vi "LEDName2Counter.vi"(10 "LED Name":string, 11 "LED Values":T1(array[cluster])) -> (3 "Counter":string)   [LabVIEW 2010, in "Settings.lvclass"]
uses:
  Settings.lvclass
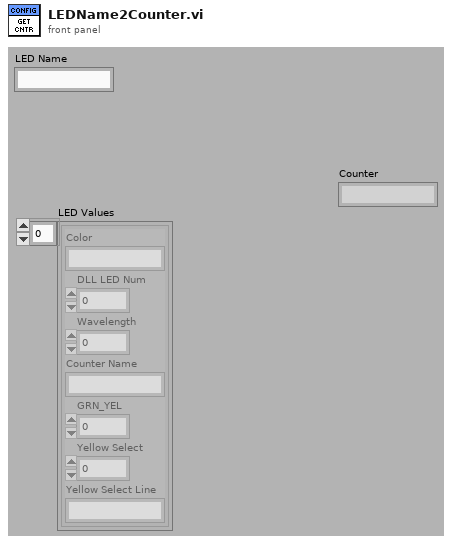
[diagram p1: front panel]
types:
  T1 = cluster{"Color":string, "DLL LED Num":i32, "Wavelength":i32, "Counter Name":string, "GRN_YEL":i32, "Yellow Select":i32, "Yellow Select Line":string}[]
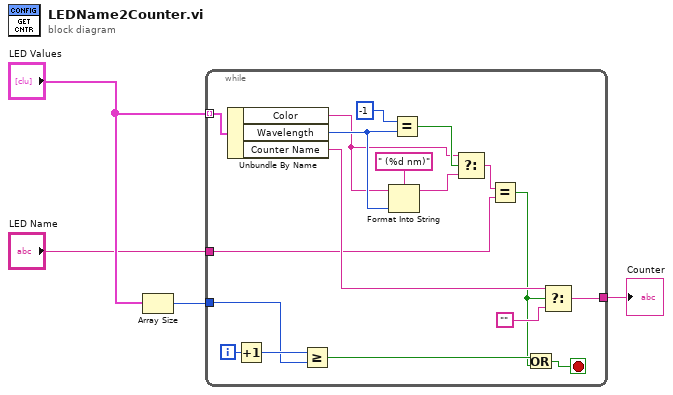
[diagram p0: block diagram]
diagram:
  n1 = Array Size(array="LED Values") -> (size(s)=w4:i32)
  n2 = while {
    tunnel: "LED Values" -> [w17] mode=indexing
    tunnel: w4 -> [w20]
    tunnel: [w16] -> w3
    tunnel: "LED Name" -> [w7]
    i -> [w22]
    stop <- w18 stop-if-true
    n3 = Unbundle By Name(w17) -> ("Color"=w9:string, "Wavelength"=w10:i32, "Counter Name"=w8:string)
    n4 = Increment(x=w22) -> (x+1=w21:i32)
    n5 = Greater Or Equal?(x=w21, y=w20) -> (x >= y?=w19:bool)
    n6 = Format Into String(format string=" (%d nm)", initial string=w9, w10) -> (resulting string=w11:string)  [unwired: 1 in, 1 out]
    n7 = Equal?(x=-1, y=w10) -> (x = y?=w12:bool)
    n8 = Select(t=w9, s=w12, f=w11) -> (s? t:f=w6:string)
    n9 = Equal?(x=w6, y=w7) -> (x = y?=w5:bool)
    n10 = Or(x=w19, y=w5) -> (x .or. y?=w18:bool)
    n11 = Select(t=w8, s=w5, f="") -> (s? t:f=w16:string)
  }
  "Counter" <- w3
